vi "Results_FromReadMethod.vi"(8 "error in (no error)":errorcluster, 11 "appended array":dbl[](array[numeric])) -> (0 "error out":errorcluster)   [LabVIEW 2017, in "WordManipulationLibrary.lvlib"]
uses:
  WordManipulationLibrary.lvlib
  MotionIO.ctl
  Read_Trajectory.ctl
panel:
  out "Feedback Info":T1
  out "Motion IO":T2
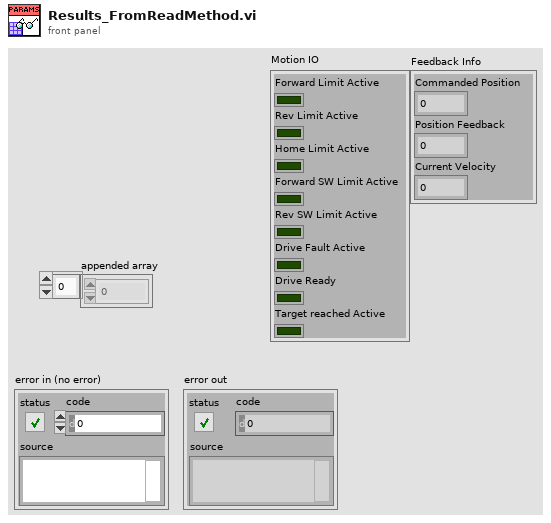
[diagram p1: front panel]
types:
  T1 = typedef "WordManipulationLibrary.lvlib/Read_Trajectory.ctl" = cluster{"Commanded Position":dbl, "Position Feedback":dbl, "Current Velocity":dbl}
  T2 = typedef "WordManipulationLibrary.lvlib/MotionIO.ctl" = cluster{"Forward Limit Active":bool, "Rev Limit Active":bool, "Home Limit Active":bool, "Forward SW Limit Active":bool, "Rev SW Limit Active":bool, "Drive Fault Active":bool, "Drive Ready":bool, "Target reached Active":bool}
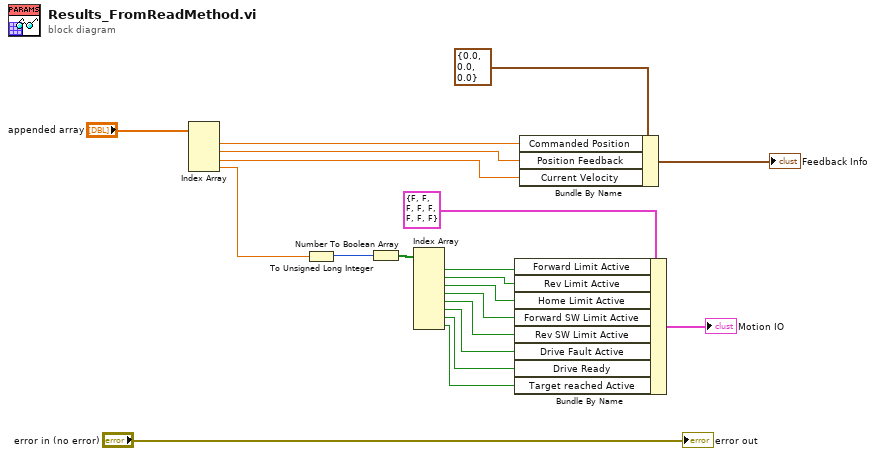
[diagram p0: block diagram]
diagram:
  n1 = Index Array(array="appended array") -> (element #1=w18:dbl, element #2=w17:dbl, element #3=w16:dbl, element #4=w14:dbl)  [unwired: 4 in]
  n2 = To Unsigned Long Integer(number=w14) -> (unsigned 32bit integer=w13:u32)
  n3 = Number To Boolean Array(number=w13) -> (Boolean array=w11:bool[])
  n4 = Index Array(array=w11) -> (element #1=w10:bool, element #2=w9:bool, element #3=w8:bool, element #4=w7:bool, element #5=w6:bool, element #6=w5:bool, element #7=w4:bool, element #8=w3:bool)  [unwired: 8 in]
  n5 = Bundle By Name(cluster=T2 {"Forward Limit Active"=FALSE, "Rev Limit Active"=FALSE, "Home Limit Active"=FALSE, "Forward SW Limit Active"=FALSE, "Rev SW Limit Active"=FALSE, "Drive Fault Active"=FALSE, "Drive Ready"=FALSE, "Target reached Active"=FALSE} ("MotionIO"), "Forward Limit Active"=w10, "Rev Limit Active"=w9, "Home Limit Active"=w8, "Forward SW Limit Active"=w7, "Rev SW Limit Active"=w6, "Drive Fault Active"=w5, "Drive Ready"=w4, "Target reached Active"=w3) -> (→"Motion IO":T2)
  n6 = Bundle By Name(cluster=T1 {"Commanded Position"=0.0, "Position Feedback"=0.0, "Current Velocity"=0.0}, "Commanded Position"=w18, "Position Feedback"=w17, "Current Velocity"=w16) -> (→"Feedback Info":T1)
  "error out" <- "error in (no error)"
